vi "Get Process Project Actions.vi"(8 "error in (no error)":errorcluster {"code" format="Error %.0f"}, 11 "VIDoc Printer In":refnum<class "VIDoc Printer.lvclass">) -> (0 "error out":errorcluster {"code" format="Error %.0f"}, 2 "Process Project Actions":T1[](array[typedef]), 3 "VIDoc Printer Out":refnum<class "VIDoc Printer.lvclass">)   [LabVIEW 2023, in "VIDoc Printer.lvlib" / "VIDoc Printer.lvclass"]
uses:
  VIDoc Printer.lvclass
  Controls/Process Project Enum.ctl
  VIDoc Printer.lvclass/VIDoc Printer.ctl
  Get Project Settings - Descriptions.vi
  Get Project Settings - Memory.vi
  Get Project Settings - Options.vi
  Get Project Settings - Symbols.vi
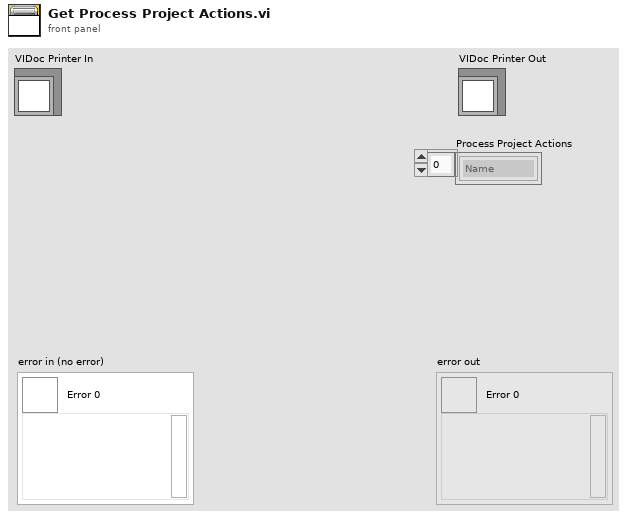
[diagram p1: front panel]
types:
  T1 = typedef "VIDoc Printer.lvlib/VIDoc Printer.lvclass/Process Project Enum.ctl" = enum16{"Name", "Description", "Memory", "Options", "Symbols"}
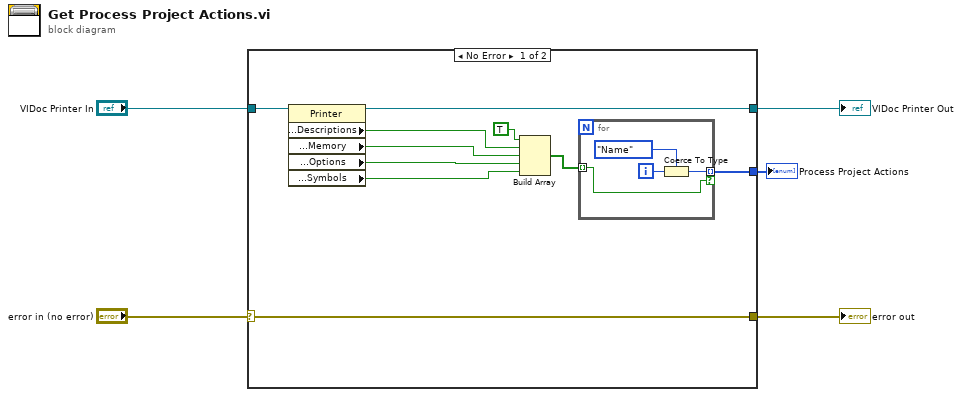
[diagram p0: block diagram]
diagram:
  n1 = case shown="No Error" "error in (no error)" {
    selector: "error in (no error)" -> [w15 w21]
    tunnel: [w15 w21] -> w4
    tunnel: [w8 w20] -> w2
    tunnel: "VIDoc Printer In" -> [w9 w20]
    tunnel: [w6 _] -> w1
    frame No Error {
      n2 = property class="Printer"(reference=w9) -> (reference out=w8:refnum<class "VIDoc Printer.lvclass">, "Properties:Settings:Projects:Descriptions"=w13:bool, "Properties:Settings:Projects:Memory"=w12:bool, "Properties:Settings:Projects:Options"=w11:bool, "Properties:Settings:Projects:Symbols"=w10:bool)  [unwired: 1 in, 1 out]
      n3 = Build Array(TRUE ("element"), w13, w12, w11, w10) -> (w7:bool[])
      n4 = for {
        tunnel: w7 -> [w16] mode=indexing
        tunnel: [w17] -> w6 mode=indexing if=w16
        i -> [w18]
        n5 = Coerce To Type(0:w18, 1:Process_Project_Enum."Name") -> (2:w17:T1)
      }
    }
    frame Error {
    }
  }
  "error out" <- w4
  "VIDoc Printer Out" <- w2
  "Process Project Actions" <- w1
